vi "Shutdown Master.vi"(8 "error in":errorcluster, 11 "Network Master in":refnum<class "Network Master.lvclass">) -> (0 "error out":errorcluster, 3 "Network Master out":refnum<class "Network Master.lvclass">)   [LabVIEW 2012, in "Network Master.lvclass"]
doc: "This provides an interface for the master to close a connection to the slave."
uses:
  Network Master.lvclass
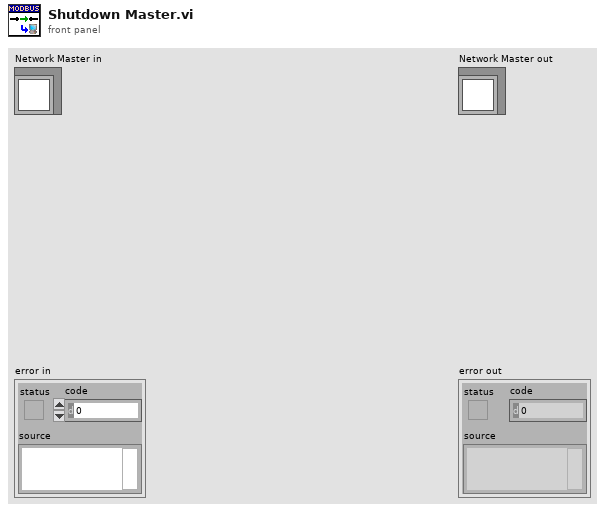
[diagram p1: front panel]
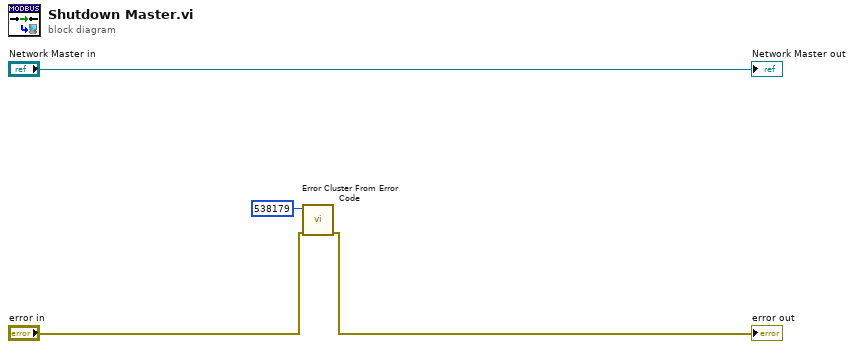
[diagram p0: block diagram]
diagram:
  n1 = call <vilib>:"Error Cluster From Error Code.vi"("error in (no error)"="error in", "error code (0)"=538179) -> ("error out"=→"error out":errorcluster)  [unwired: 7 in]
  "Network Master out" <- "Network Master in"
